vi "waitOnConsoleStart.vi"(8 "error in (no error)":errorcluster, 11 "Handler.UserEvent.Console in":refnum<class "Handler.UserEvent.Console.lvclass">) -> (0 "error out":errorcluster, 3 "Handler.UserEvent.Console out":refnum<class "Handler.UserEvent.Console.lvclass">)   [LabVIEW 2017, in "Error Log.lvlib" / "Handler.UserEvent.Console.lvclass"]
uses:
  Handler.UserEvent.Console.lvclass
  Handler.UserEvent.Console.lvclass/Handler.UserEvent.Console.ctl
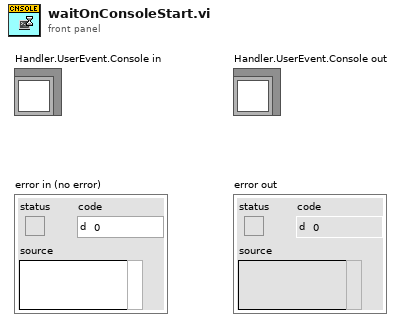
[diagram p1: front panel]
types:
  T1 = enum32{"Bad", "Idle", "Run top level", "Running"}
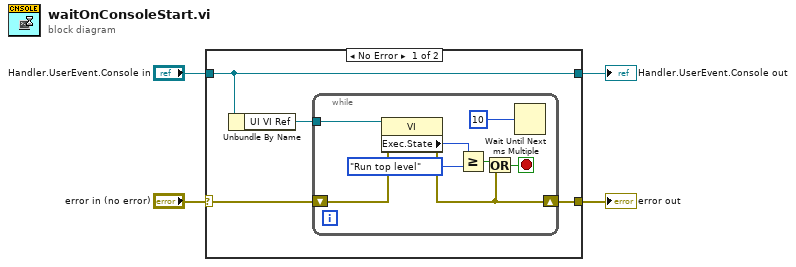
[diagram p0: block diagram]
diagram:
  n1 = case shown="No Error" "error in (no error)" {
    selector: "error in (no error)" -> [w6 w18]
    tunnel: [w5 w18] -> w3
    tunnel: [w8 w17] -> w1
    tunnel: "Handler.UserEvent.Console in" -> [w8 w17]
    frame No Error {
      n2 = Unbundle By Name(w8) -> ("UI VI Ref"=w7:refnum<vi>)
      n3 = while {
        tunnel: w7 -> [w16]
        shift-right: [w9] -> w5
        shift-left: w6 -> [w11]
        stop <- w10 stop-if-true
        n4 = property class="VI"(reference=w16, error in=w11) -> (error out=w9:errorcluster, "Exec.State"=w15:T1)  [unwired: 1 out]
        n5 = Greater Or Equal?(x=w15, y=T1."Run top level") -> (x >= y?=w13:bool)
        n6 = Or(x=w13, y=w9) -> (x .or. y?=w10:bool)
        n7 = Wait Until Next ms Multiple(millisecond multiple=u32 10) -> ()  [unwired: 1 out]
      }
    }
    frame Error {
    }
  }
  "error out" <- w3
  "Handler.UserEvent.Console out" <- w1
